vi "get pid.vi"() -> (0 "PID":u32)   [LabVIEW 2017]
uses:
  kernel32.dll
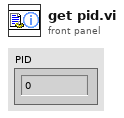
[diagram p1: front panel]
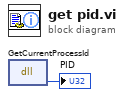
[diagram p0: block diagram]
diagram:
  n1 = dll-call lib="kernel32.dll" fn="GetCurrentProcessId"() -> ("return type"=→"PID":u32)  [unwired: 3 in, 2 out]
